vi "换算-时间差至日时分秒.vi"(7 "时长模式":T1(ring), 10 "时间1":timestamp, 11 "时间2":timestamp) -> (3 "时长":cluster{"天":i32, "时":i32, "分":i32, "秒":i32}, 4 "时长 s":dbl)   [LabVIEW 2017]
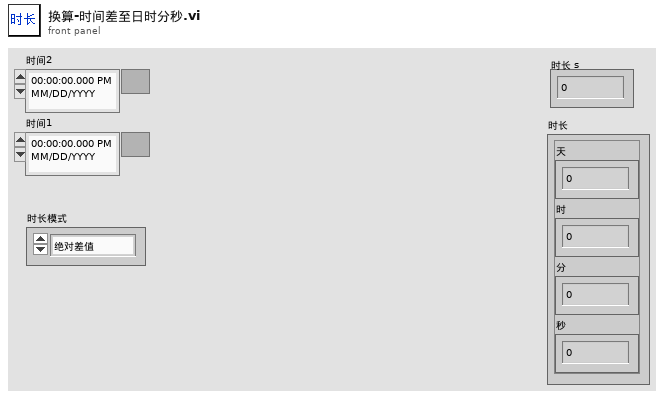
[diagram p1: front panel]
types:
  T1 = enum16{"绝对差值", "取整+1s", "取整+1m", "取整+1h", "取整+1d"}
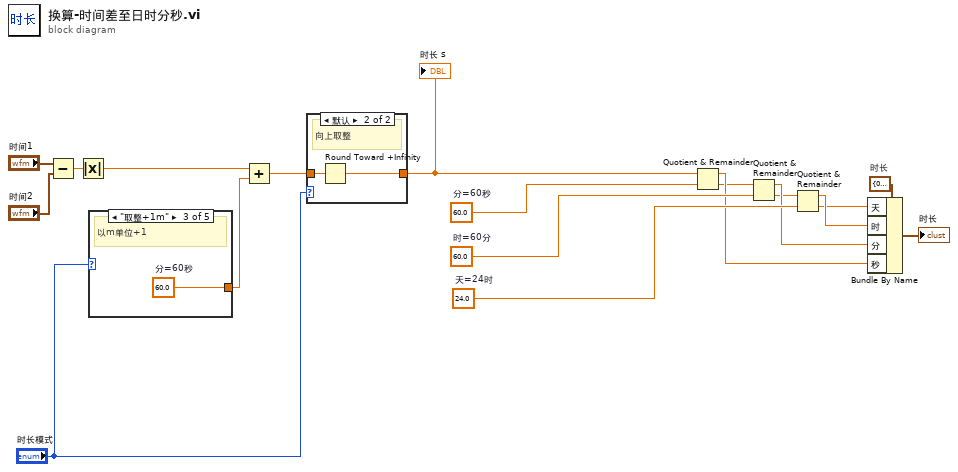
[diagram p0: block diagram]
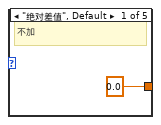
[diagram p3: hidden frame]
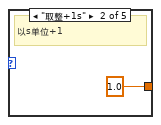
[diagram p4: hidden frame]
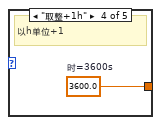
[diagram p5: hidden frame]
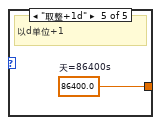
[diagram p6: hidden frame]
diagram:
  w13 = cluster{"天":i32, "时":i32, "分":i32, "秒":i32} {"天"=0, "时"=0, "分"=0, "秒"=0}  # 时长
  w14 = 24.0  # 天=24时
  w15 = 60.0  # 时=60分
  w16 = 60.0  # 分=60秒
  n1 = Subtract(x="时间1", y="时间2") -> (x-y=w18:dbl)
  n2 = Absolute Value(x=w18) -> (abs(x)=w5:dbl)
  n3 = case shown="\"取整+1m\"" "时长模式" {
    tunnel: [0.0 1.0 w22 w23 w24] -> w1
    frame "绝对差值", Default {
      # "不加"
    }
    frame "取整+1s" {
      # "以s单位+1"
    }
    frame "取整+1m" {
      w22 = 60.0  # 分=60秒
      # "以m单位+1"
    }
    frame "取整+1h" {
      w23 = 3600.0  # 时=3600s
      # "以h单位+1"
    }
    frame "取整+1d" {
      w24 = 86400.0  # 天=86400s
      # "以d单位+1"
    }
  }
  n4 = Add(x=w5, y=w1) -> (x+y=w3:dbl)
  n5 = case shown="默认" "时长模式" {
    tunnel: w3 -> [w25 w27]
    tunnel: [w25 w26] -> w2
    frame "绝对差值" {
      # "直接对二者求差"
    }
    frame Default {
      # "向上取整"
      n6 = Round Toward +Infinity(x=w27) -> (ceil(x): smallest int >= x=w26:dbl)
    }
  }
  "时长 s" <- w2
  n7 = Quotient & Remainder(x=w2, y=w16) -> (x-y*floor(x/y)=w12:dbl, floor(x/y)=w10:dbl)
  n8 = Quotient & Remainder(x=w10, y=w15) -> (x-y*floor(x/y)=w9:dbl, floor(x/y)=w8:dbl)
  n9 = Quotient & Remainder(x=w8, y=w14) -> (x-y*floor(x/y)=w7:dbl, floor(x/y)=w6:dbl)
  n10 = Bundle By Name(cluster=w13, "天"=w6, "时"=w7, "分"=w9, "秒"=w12) -> (→"时长":cluster{"天":i32, "时":i32, "分":i32, "秒":i32})
